vi "Terminal-Core-StorageModule.vi"(8 "error in":errorcluster, 9 "ErrorQRef":refnum<queue>, 10 "DataQRef":refnum<queue>) -> (0 "错误输出":errorcluster)   [LabVIEW 2014]
panel:
  in  "开关":bool=TRUE
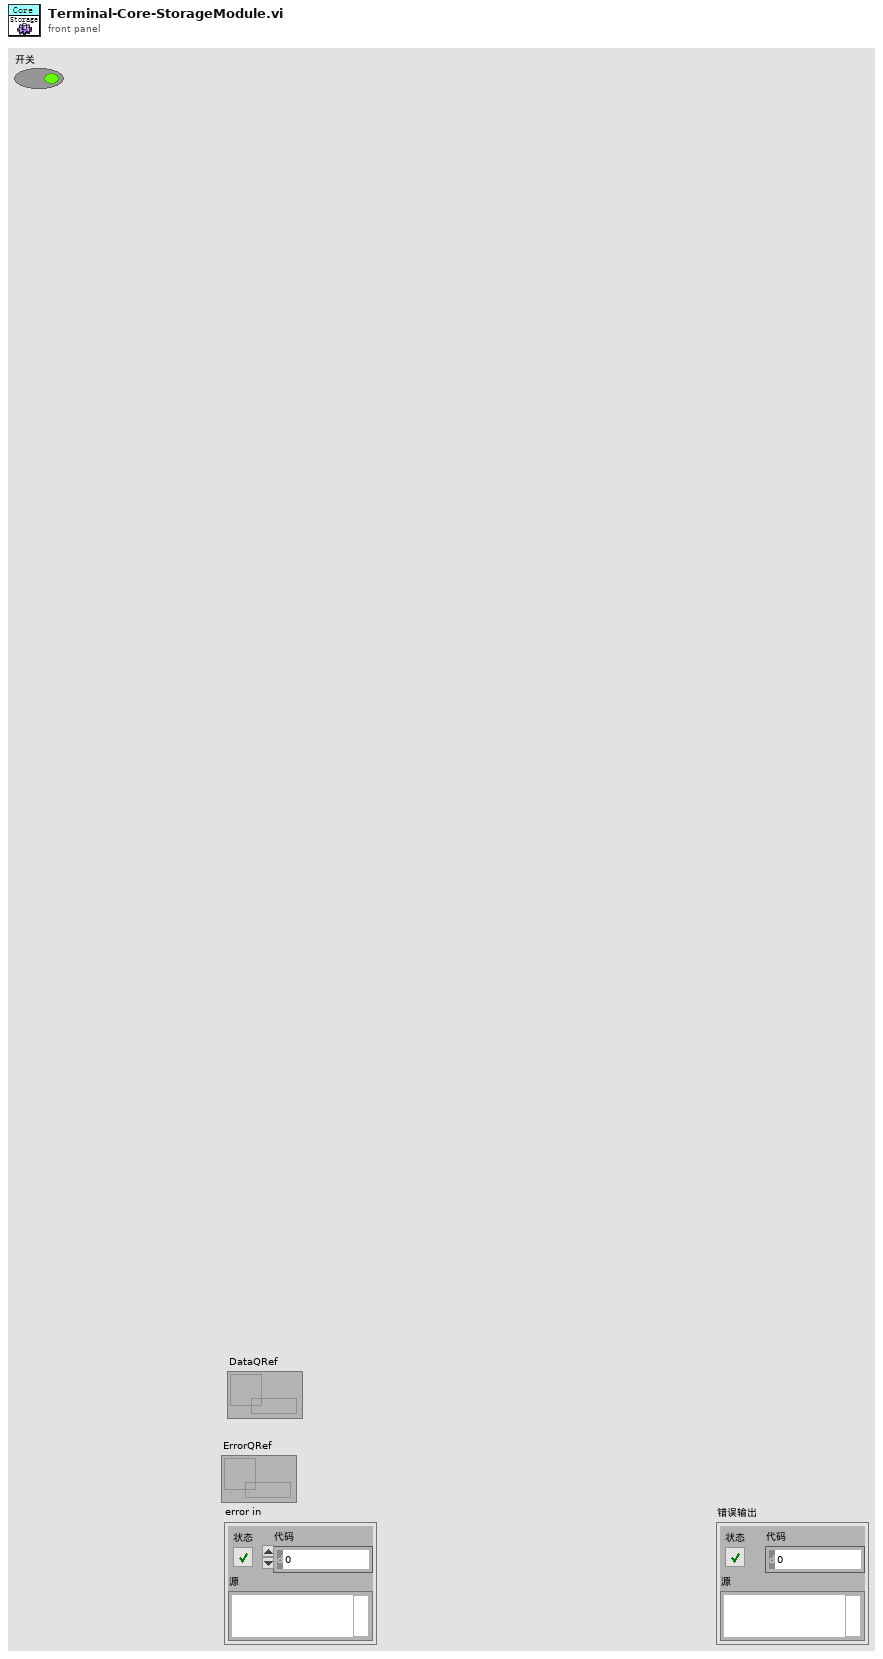
[diagram p1: front panel]
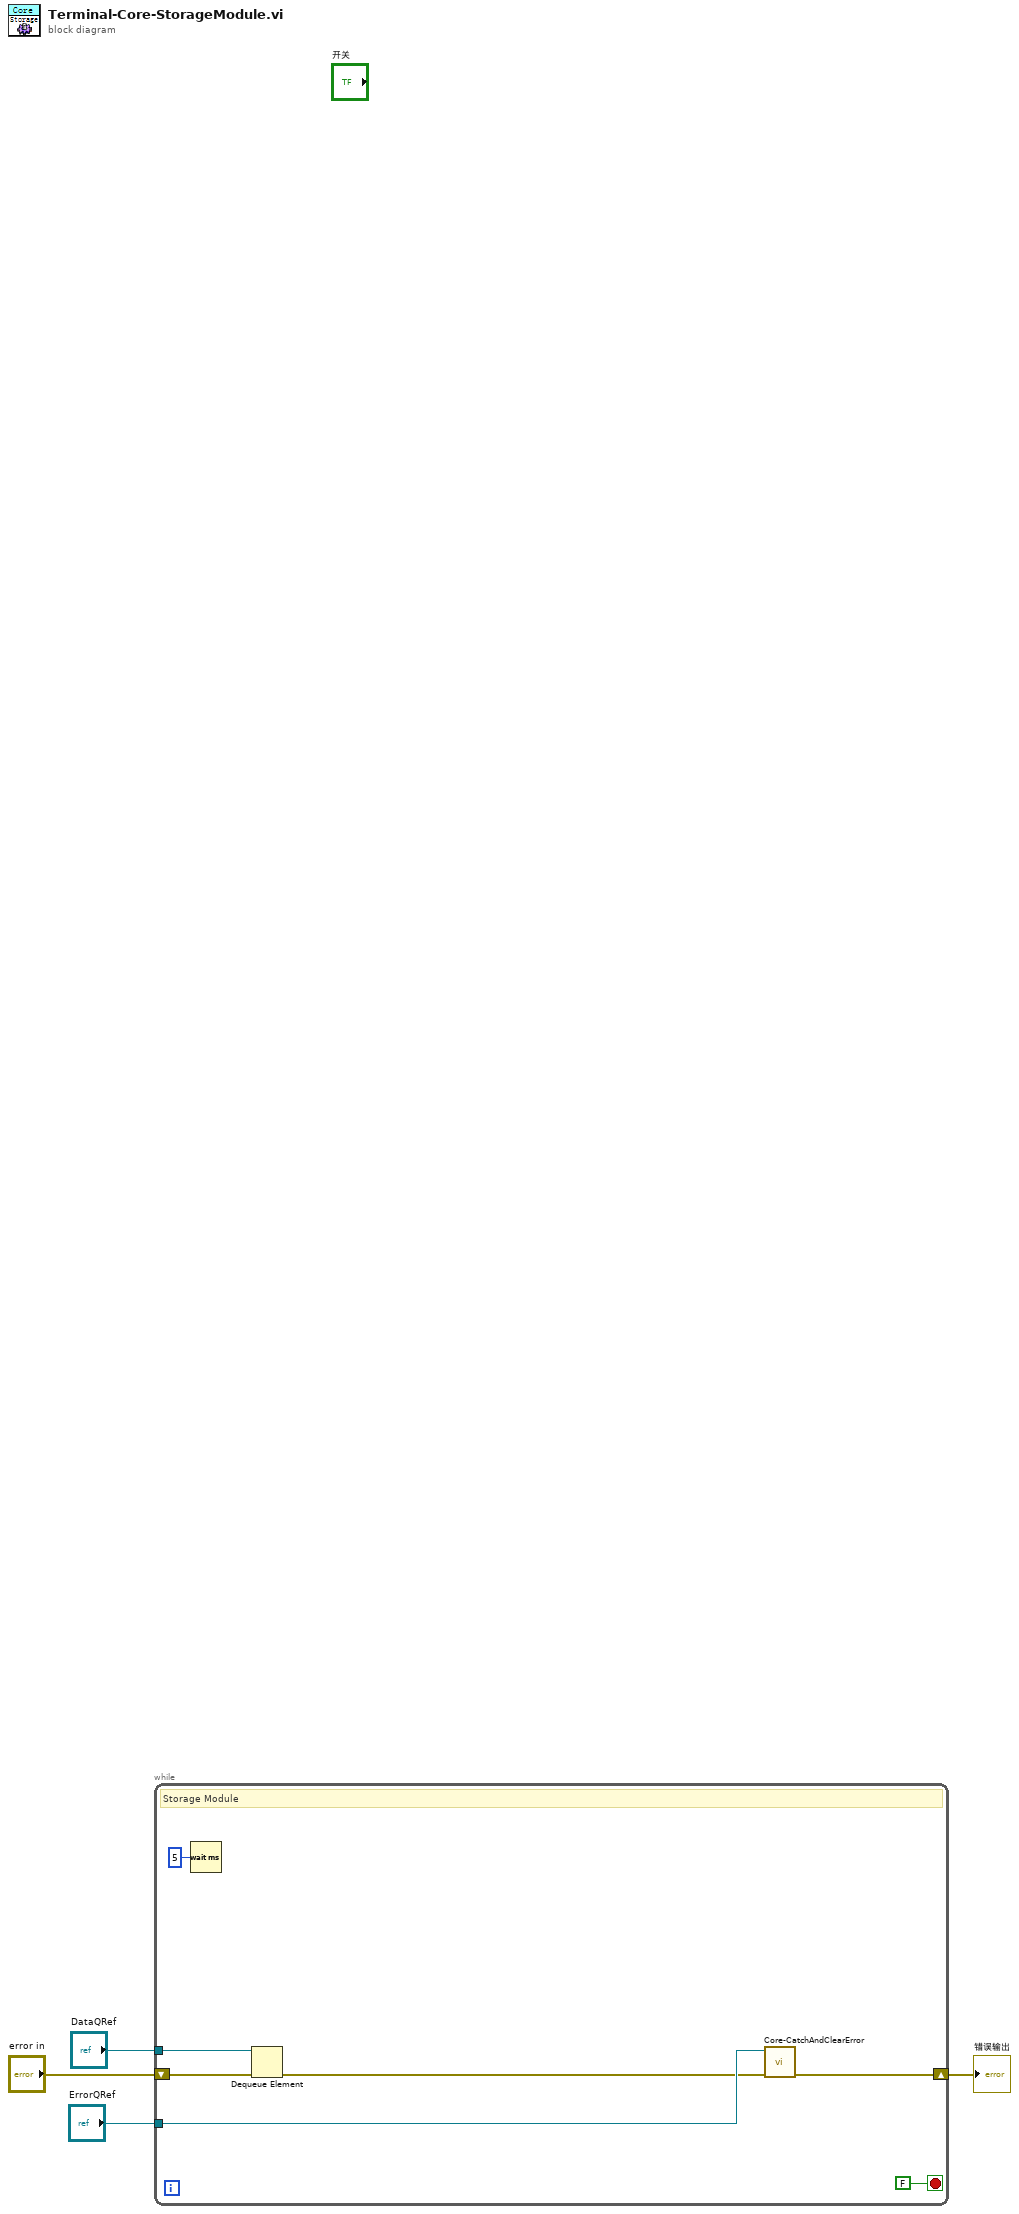
[diagram p0: block diagram]
diagram:
  n1 = while {
    tunnel: "DataQRef" -> [w10]
    shift-right: [w9] -> w2
    shift-left: "error in" -> [w7]
    tunnel: "ErrorQRef" -> [w8]
    stop <- FALSE stop-if-true
    # "Storage Module"
    n2 = Wait (ms)(milliseconds to wait=u32 5 ("等待时间（毫秒）")) -> ()  [unwired: 1 out]
    n3 = Dequeue Element(queue=w10, error in (no error)=w7) -> (error out=w6:errorcluster)  [unwired: 1 in, 3 out]
    n4 = call "Core-CatchAndClearError.vi"("error in (no error)"=w6, "ErrorQ"=w8) -> ("error out"=w9:errorcluster)  [unwired: 7 in]
  }
  "错误输出" <- w2
